vi "Required String Buffer Size (Transfer).vi"(8 "error in (no error)":errorcluster, 11 "Transfer Configuration in":T1 {"channel blocks"."string descriptor"."buffer offset" format="%d bytes"; "channel blocks"."engine descriptor"."buffer offset" format="%d bytes"}) -> (0 "error out":errorcluster, 2 "required string buffer size":u64 format="%d bytes", 3 "Transfer Configuration out":T1 {"channel blocks"."string descriptor"."buffer offset" format="%d bytes"; "channel blocks"."engine descriptor"."buffer offset" format="%d bytes"})   [LabVIEW 2017, in "DSF Core.lvlib"]
uses:
  DSF Core.lvlib
  Controls/DSF Engine Transfer Configuration.ctl
  Controls/DSF Byte Order.ctl
  Controls/DSF Engine Channel Configuration.ctl
  Controls/DSF Channel Buffer Descriptor.ctl
  Controls/DSF Data Type.ctl
  Controls/DSF Settings Info.ctl
  Shared/VIs/Sizeof.vi
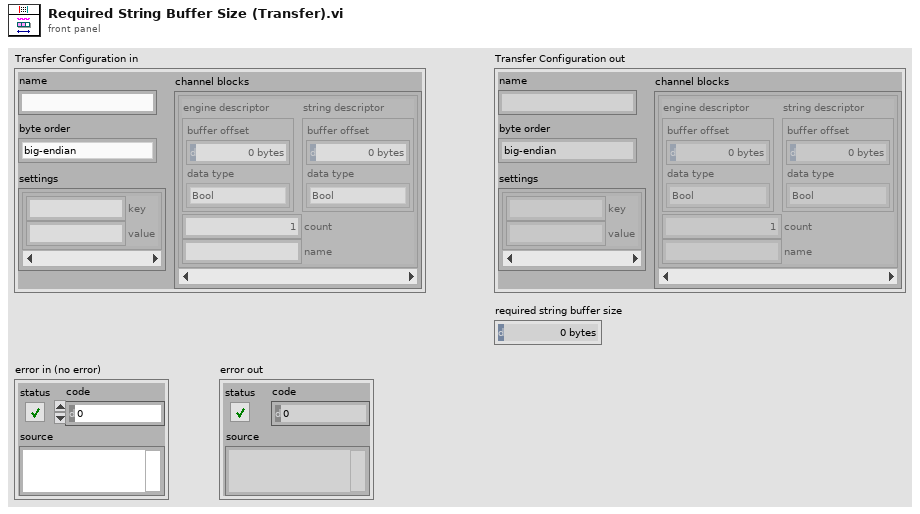
[diagram p1: front panel]
types:
  T1 = typedef "DSF Core.lvlib/DSF Engine Transfer Configuration.ctl" = cluster{"name":string, "byte order":T2, "channel blocks":T3[], "settings":T6}
  T2 = typedef "DSF Core.lvlib/DSF Byte Order.ctl" = enum8{"big-endian", "little-endian"}
  T3 = typedef "DSF Core.lvlib/DSF Engine Channel Configuration.ctl" = cluster{"engine descriptor":T4, "string descriptor":T4, "count":u64, "name":string}
  T4 = typedef "DSF Core.lvlib/DSF Channel Buffer Descriptor.ctl" = cluster{"buffer offset":u64, "data type":T5}
  T5 = typedef "DSF Core.lvlib/DSF Data Type.ctl" = enum8{"Bool", "SGL", "DBL", "I8", "I16", "I32", "I64", "U8", "U16", "U32", "U64"}
  T6 = typedef "DSF Core.lvlib/DSF Settings Info.ctl" = cluster{"key":string, "value":string}[]
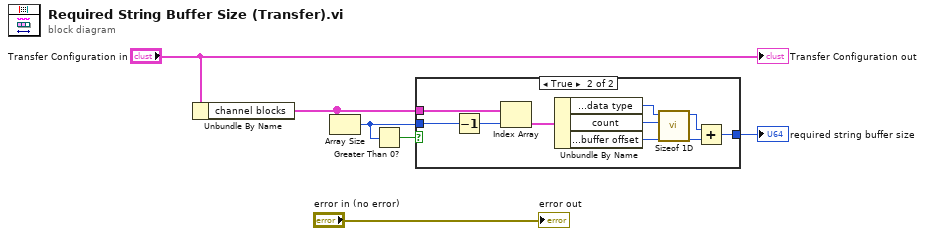
[diagram p0: block diagram]
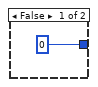
[diagram p2: hidden frame]
diagram:
  n1 = Unbundle By Name("Transfer Configuration in") -> ("channel blocks"=w3:T3[])
  n2 = Array Size(array=w3) -> (size(s)=w6:i32)
  n3 = Greater Than 0?(x=w6) -> (x > 0?=w5:bool)
  n4 = case shown="True" w5 {
    tunnel: w6 -> [_ w16]
    tunnel: w3 -> [_ w15]
    tunnel: [u64 0 w8] -> w4
    frame False {
    }
    frame True {
      n5 = Decrement(x=w16) -> (x-1=w14:i32)
      n6 = Index Array(array=w15, index=w14) -> (element=w13:T3)
      n7 = Unbundle By Name(w13) -> ("string descriptor.data type"=w12:T5, "count"=w11:u64, "string descriptor.buffer offset"=w10:u64)
      n8 = call "Sizeof 1D.vi"("count"=w11, "data type"=w12) -> ("size in bytes"=w9:u64)  [unwired: 9 in]
      n9 = Add(x=w9, y=w10) -> (x+y=w8:u64)
    }
  }
  "required string buffer size" <- w4
  "Transfer Configuration out" <- "Transfer Configuration in"
  "error out" <- "error in (no error)"
